vi "Get Path Node VI.vi"(8 "error in (no error)":errorcluster, 11 "Node ref in":refnum<k20>) -> (0 "error out":errorcluster, 1 "Found ?":bool, 2 "VI Name out":string, 3 "Node ref out":refnum<k20>)   [LabVIEW 2018, in ".LVLIBP CD XML Updater.lvlib" / "Project XML Editor.lvclass"]
uses:
  Project XML Editor.lvclass
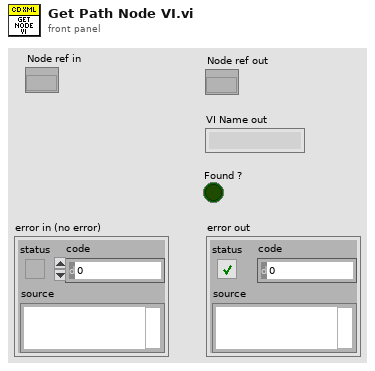
[diagram p1: front panel]
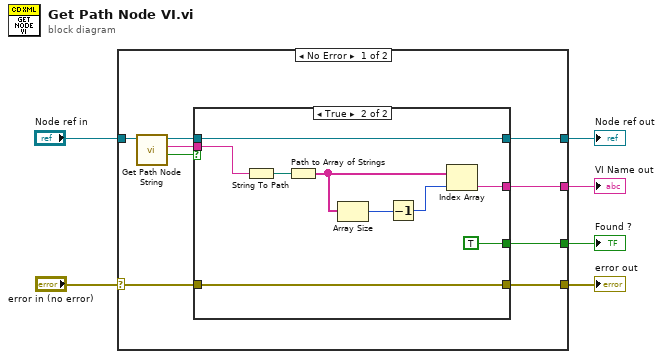
[diagram p0: block diagram]
diagram:
  n1 = case shown="No Error" "error in (no error)" {
    selector: "error in (no error)" -> [w10 w30]
    tunnel: "Node ref in" -> [w15 w29]
    tunnel: [w9 w30] -> w4
    tunnel: [w12 w29] -> w3
    tunnel: [w8 _] -> w2
    tunnel: [w7 _] -> w1
    frame No Error {
      n2 = call "Get Path Node String.vi"("Node ref in"=w15) -> ("Found ?"=w14:bool, "Path out"=w11:string, "Node ref out"=w13:refnum<k20>)  [unwired: 7 in, 1 out]
      n3 = case shown="True" w14 {
        selector: w14 -> [w16 _]
        tunnel: w11 -> [w18 w28]
        tunnel: [w18 w25] -> w7
        tunnel: w13 -> [w19 w24]
        tunnel: [w19 w24] -> w12
        tunnel: w10 -> [w17 w23]
        tunnel: [w17 w23] -> w9
        tunnel: [w16 TRUE] -> w8
        frame False {
        }
        frame True {
          n4 = String To Path(string=w28) -> (path=w27:path)
          n5 = Path to Array of Strings(0:w27) -> (2:w26:string[])  [unwired: 1 out]
          n6 = Array Size(array=w26) -> (size(s)=w22:i32)
          n7 = Decrement(x=w22) -> (x-1=w21:i32)
          n8 = Index Array(array=w26, index=w21) -> (element=w25:string)
        }
      }
    }
    frame Error {
    }
  }
  "VI Name out" <- w1
  "error out" <- w4
  "Node ref out" <- w3
  "Found ?" <- w2
